vi "input_output_constants.vi"() -> (0 "mag inputs":tag[](array[tag]), 1 "heat outputs":refnum<k21>[](array[refnum]), 2 "heat inputs":tag[](array[tag]), 3 "labels":string[](array[string]))   [LabVIEW 2015]
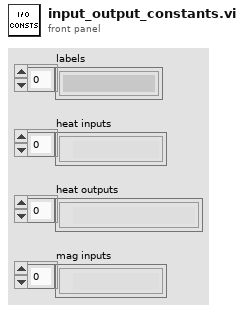
[diagram p1: front panel]
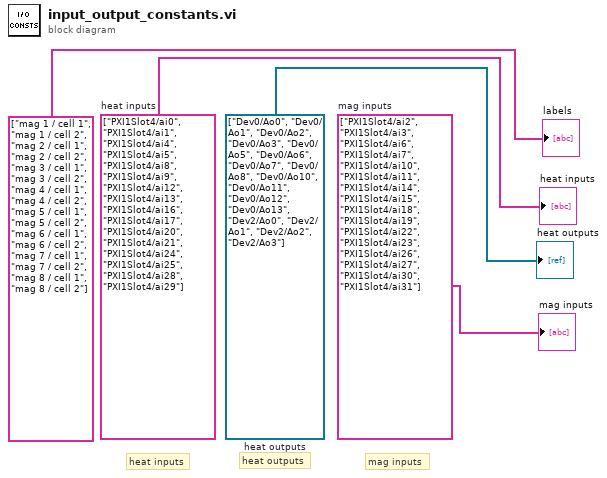
[diagram p0: block diagram]
diagram:
  w2 = tag[] ["PXI1Slot4/ai2", "PXI1Slot4/ai3", "PXI1Slot4/ai6", "PXI1Slot4/ai7", "PXI1Slot4/ai10", "PXI1Slot4/ai11", "PXI1Slot4/ai14", "PXI1Slot4/ai15", "PXI1Slot4/ai18", "PXI1Slot4/ai19", "PXI1Slot4/ai22", "PXI1Slot4/ai23", "PXI1Slot4/ai26", "PXI1Slot4/ai27", "PXI1Slot4/ai30", "PXI1Slot4/ai31"]  # mag inputs
  w1 = refnum<k21>[] ["Dev0/Ao0", "Dev0/Ao1", "Dev0/Ao2", "Dev0/Ao3", "Dev0/Ao5", "Dev0/Ao6", "Dev0/Ao7", "Dev0/Ao8", "Dev0/Ao10", "Dev0/Ao11", "Dev0/Ao12", "Dev0/Ao13", "Dev2/Ao0", "Dev2/Ao1", "Dev2/Ao2", "Dev2/Ao3"]  # heat outputs
  w3 = tag[] ["PXI1Slot4/ai0", "PXI1Slot4/ai1", "PXI1Slot4/ai4", "PXI1Slot4/ai5", "PXI1Slot4/ai8", "PXI1Slot4/ai9", "PXI1Slot4/ai12", "PXI1Slot4/ai13", "PXI1Slot4/ai16", "PXI1Slot4/ai17", "PXI1Slot4/ai20", "PXI1Slot4/ai21", "PXI1Slot4/ai24", "PXI1Slot4/ai25", "PXI1Slot4/ai28", "PXI1Slot4/ai29"]  # heat inputs
  # "mag inputs"
  # "heat outputs"
  # "heat inputs"
  "labels" <- string[] ["mag 1 / cell 1", "mag 1 / cell 2", "mag 2 / cell 1", "mag 2 / cell 2", "mag 3 / cell 1", "mag 3 / cell 2", "mag 4 / cell 1", "mag 4 / cell 2", "mag 5 / cell 1", "mag 5 / cell 2", "mag 6 / cell 1", "mag 6 / cell 2", "mag 7 / cell 1", "mag 7 / cell 2", "mag 8 / cell 1", "mag 8 / cell 2"]
  "heat inputs" <- w3
  "mag inputs" <- w2
  "heat outputs" <- w1
